vi "List git conflicted files.vi"() -> (0 "error out":errorcluster, 3 "conflicted files list":string[](array[string]))   [LabVIEW 2022 SP3]
panel:
  out "size(s)":i32
  in  "ein":errorcluster
  out "standard error":string
  out "return code":i32
  out "standard output":string
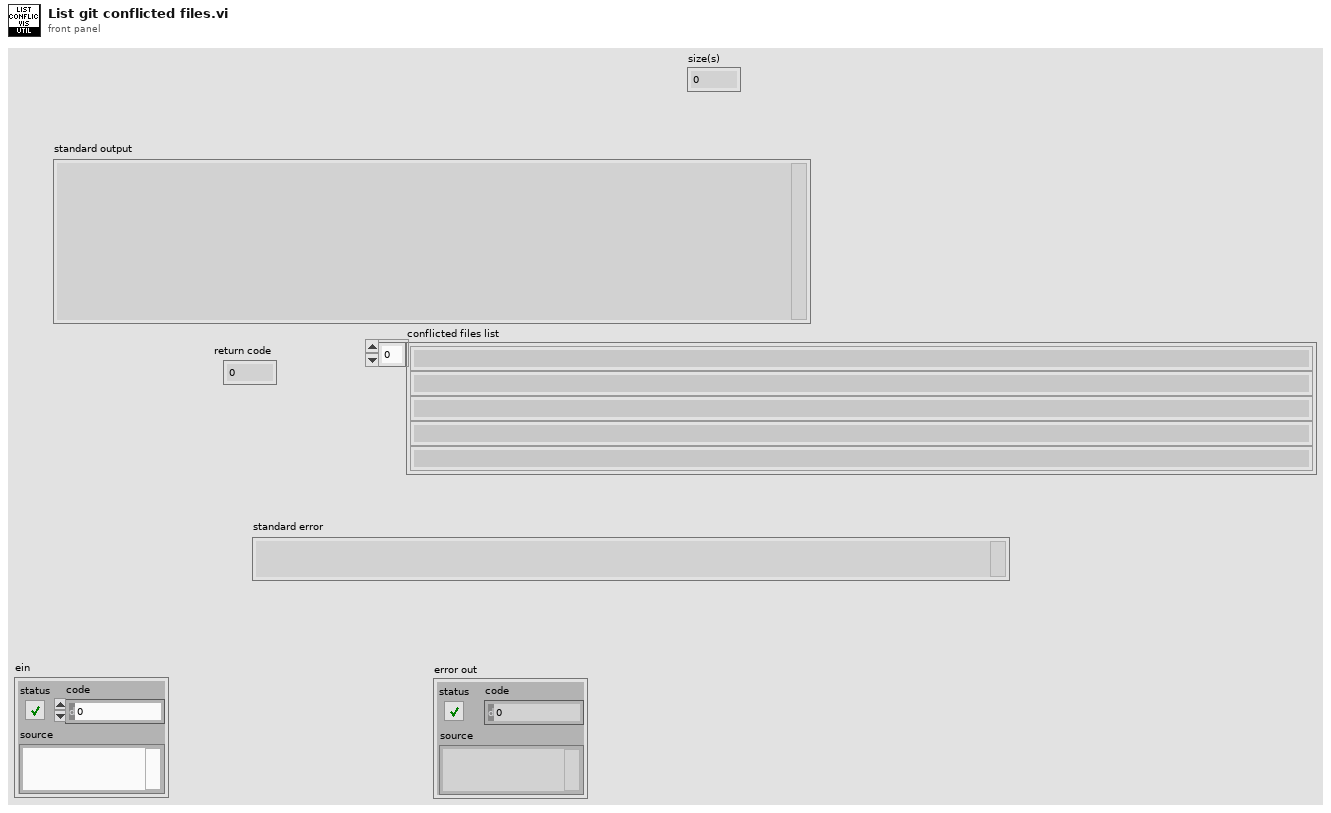
[diagram p1: front panel]
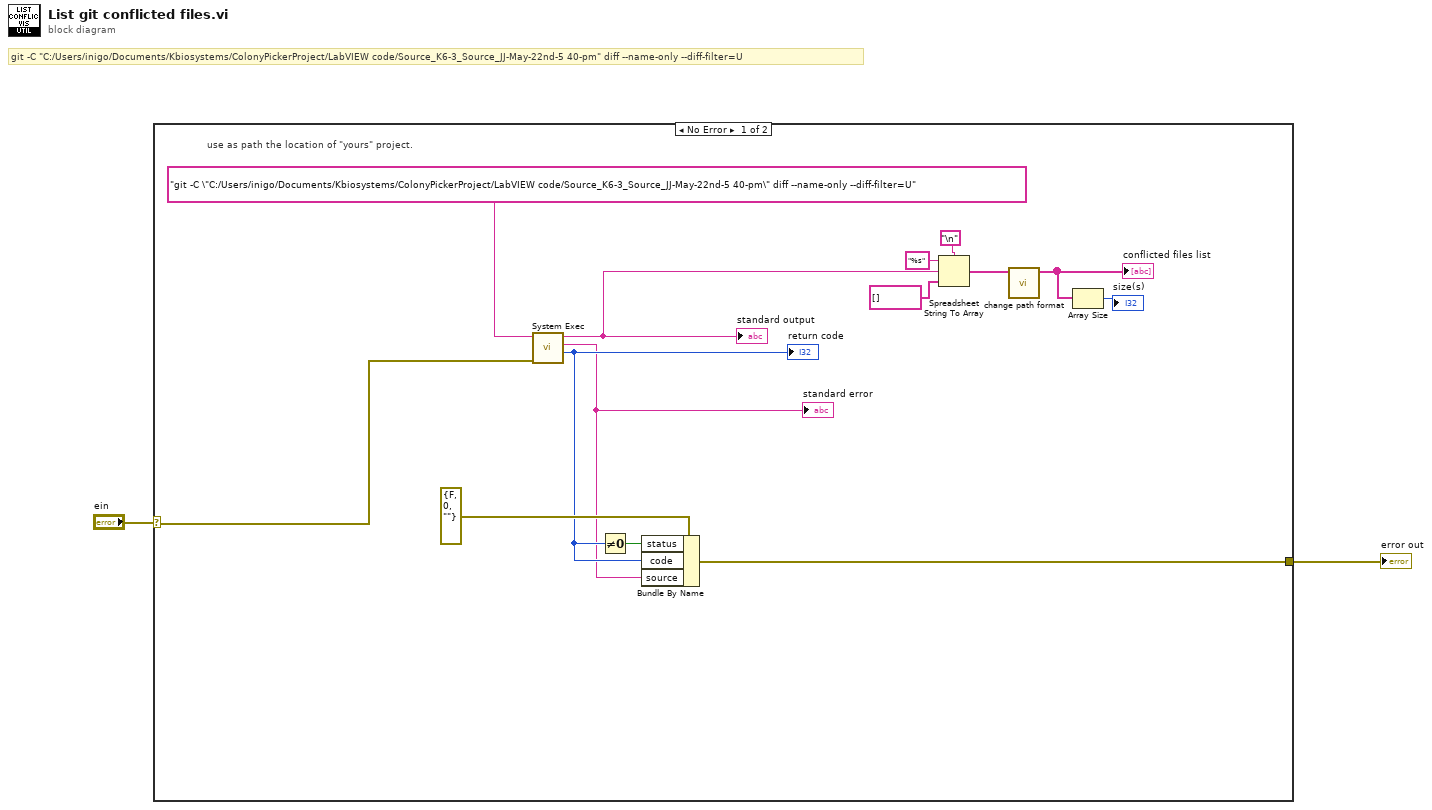
[diagram p0: block diagram]
diagram:
  # "git -C \"C:/Users/inigo/Documents/Kbiosystems/ColonyPickerProject/LabVIEW code/Source_K6-3_Source_JJ-May-22nd-5 40-pm\" diff --name-only --diff-filter=U"
  n1 = case shown="No Error" "ein" {
    selector: "ein" -> [w6 w17]
    tunnel: [w7 w17] -> w2
    frame No Error {
      # "use as path the location of \"yours\" project."
      n2 = call <vilib>:"System Exec.vi"("error in (no error)"=w6, "command line"="git -C \"C:/Users/inigo/Documents/Kbiosystems/ColonyPickerProject/LabVIEW code/Source_K6-3_Source_JJ-May-22nd-5 40-pm\" diff --name-only --diff-filter=U") -> ("return code"=w9:i32, "standard error"=w8:string, "standard output"=w14:string)  [unwired: 6 in, 1 out]
      "standard output" <- w14
      "return code" <- w9
      "standard error" <- w8
      n3 = Not Equal To 0?(x=w9) -> (x != 0?=w10:bool)
      n4 = Bundle By Name(cluster=errorcluster {"status"=FALSE, "code"=0, "source"=""} ("error in (no error)"), "status"=w10, "code"=w9, "source"=w8) -> (w7:errorcluster)
      n5 = Spreadsheet String To Array(delimiter (Tab)="\n", format string="%s", spreadsheet string=w14, array type (2D Dbl)=string[] []) -> (array=w5:string[])
      n6 = call "change path format.vi"("conflicted files list in"=w5) -> ("conflicted files list out"=w4:string[])  [unwired: 10 in]
      "conflicted files list" <- w4
      n7 = Array Size(array=w4) -> (size(s)=→"size(s)":i32)
    }
    frame Error {
    }
  }
  "error out" <- w2
